vi "Write.vi"(8 "error in":errorcluster, 10 "MessageBuffer":T1, 11 "Channel":u16) -> (0 "error out":errorcluster, 2 "MessageBuffer out":T1, 3 "Channel out":u16, 5 "function return":u32)   [LabVIEW 2025, in "PCAN API.lvlib"]
doc: "This VI is used for writting a CAN message with decoding errors from function return."
uses:
  PCAN API.lvlib
  PCAN2023/PCAN2023.lvlib
  <vilib>/Utility/file.llb/Write Delimited Spreadsheet (string).vi
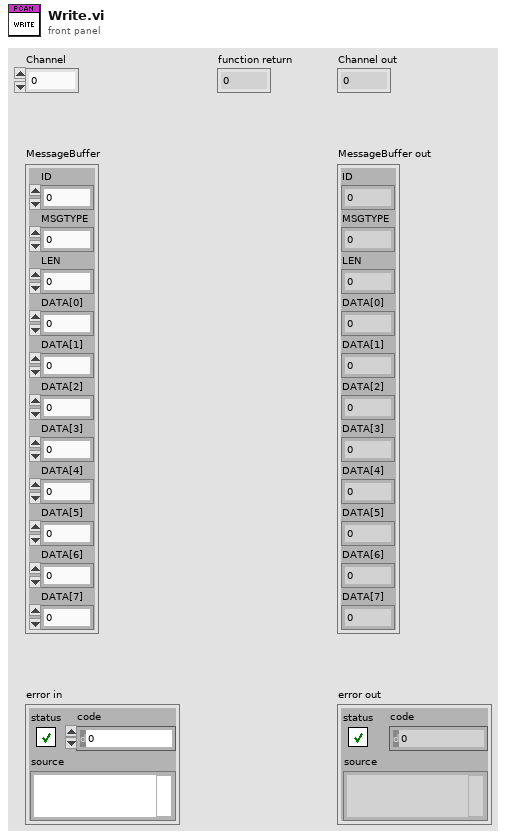
[diagram p1: front panel]
types:
  T1 = cluster{"ID":u32, "MSGTYPE":u8, "LEN":u8, "DATA[0]":u8, "DATA[1]":u8, "DATA[2]":u8, "DATA[3]":u8, "DATA[4]":u8, "DATA[5]":u8, "DATA[6]":u8, "DATA[7]":u8}
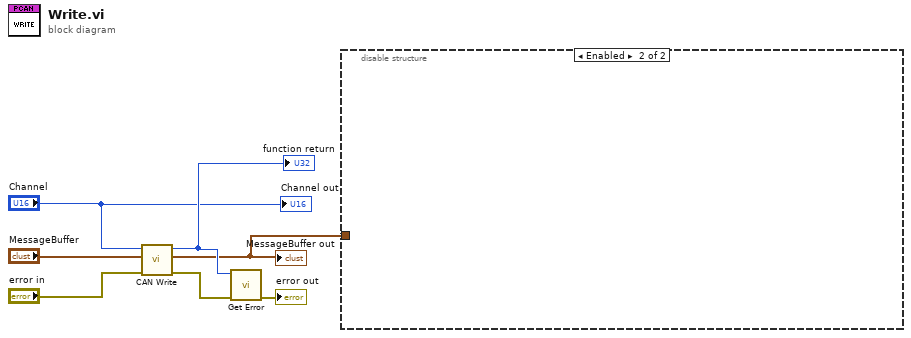
[diagram p0: block diagram]
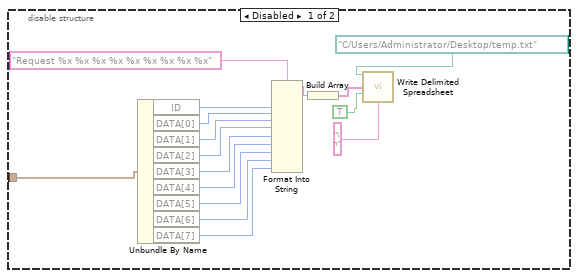
[diagram p2: hidden frame]
diagram:
  n1 = call "CAN Write.vi"("error in (no error)"="error in", "MessageBuffer"="MessageBuffer", "Channel"="Channel") -> ("error out"=w5:errorcluster, "MessageBuffer out"=w1:T1, "function return"=w3:u32)  [unwired: 5 in, 1 out]
  "function return" <- w3
  "MessageBuffer out" <- w1
  n2 = call "Get Error.vi"("error in (no error)"=w5, "function return"=w3) -> ("error out"=→"error out":errorcluster)  [unwired: 9 in]
  n3 = disable-structure shown="Enabled" {
    disable-tunnel: w1 -> [w23 _]
    frame Disabled {
      n4 = Unbundle By Name(w23) -> ("ID"=w21:u32, "DATA[0]"=w20:u8, "DATA[1]"=w19:u8, "DATA[2]"=w18:u8, "DATA[3]"=w17:u8, "DATA[4]"=w16:u8, "DATA[5]"=w15:u8, "DATA[6]"=w14:u8, "DATA[7]"=w13:u8)
      n5 = Format Into String(format string="Request %x %x %x %x %x %x %x %x %x", w21, w20, w19, w18, w17, w16, w15, w14, w13) -> (resulting string=w9:string)  [unwired: 2 in, 1 out]
      n6 = Build Array(w9) -> (w8:string[])
      n7 = call-poly <vilib>:"Write Delimited Spreadsheet.vi"("file path (dialog if empty)"=path "C:/Users/Administrator/Desktop/temp.txt", "1D data"=w8, "append to file? (new file:F)"=TRUE, "delimiter (\\t)"="\n" ("delimiter (\\t)")) -> ()  [unwired: 10 in, 2 out]
    }
    frame Enabled {
    }
  }
  "Channel out" <- "Channel"
